vi "Measurement UI.vi"() -> ()   [LabVIEW 2021, in "Ramp-Up Time_PMIC_UI.lvlib"]
uses:
  Ramp-Up Time_PMIC_UI.lvlib
panel:
  in  "MeasGraphs":T1(tab)
  out "SourceVoltageV/STimeGraph":waveform(dbl)(graph) caption="Load Transient"
  in  "SourceOutput Voltage v/s Time":string="SOURCE VOLTAGE vs TIME"
  out "OutputVoltageV/STimeGraph":waveform(dbl)(graph) caption="Load Transient"
  in  "LoadOutput Voltage v/s Time":string="LOAD VOLTAGE vs TIME"
  out "ScopeAmplitudeV/STime":waveform(dbl)(graph) caption="Load Transient"
  in  "ScopeOutput Voltage v/s Time":string="SCOPE AMPLITUDE vs TIME"
  out "Ramp stop time":dbl
  out "Ramp start time":dbl
  out "Ramp stop voltage level":dbl
  out "Ramp start voltage level":dbl
  out "Actual ramp rate":dbl
  out "Scope amplitude dt":dbl
  out "Scope amplitudes":dbl[](array[numeric])
  out "Load voltages":dbl[](array[numeric])
  out "Load voltage dt":dbl
  out "Source voltages":dbl[](array[numeric])
  out "Source voltage dt":dbl
  in  "Load resource name":string
  in  "Scope resource name":string
  in  "Source resource name":string
  in  "Source transient response":i32(ring)=1042 items=["Slow"=1041, "Normal"=1038, "Fast"=1039, "Custom"=1042]
  out "MeasTable":string[][](table)
  in  "MeasConfigurations":T2(tab)=enum."Load Config"
  in  "Source sense":i32(ring)=1009 caption="SENSE" items=["Local"=1008, "Remote"=1009]
  in  "Source ramp stop percentage(%)":dbl=90.0 caption="STOP RAMP MEASUREMENT" format="%#_6p%"
  in  "Source ramp start percentage(%)":dbl=10.0 caption="START RAMP MEASUREMENT" format="%#_6p%"
  in  "Source voltatge V2 time":dbl=0.005 caption="TIME for V1" format="%#_6ps"
  in  "Source voltage V1 time":dbl=0.005 caption="TIME for V1" format="%#_6ps"
  in  "Source voltage ramp rate":dbl=50000.0 caption="VOLTAGE RAMP RATE LIMIT" format="%#_6pV/s"
  in  "Source maximum power":dbl=300.0 caption="MAXIMUM POWER" format="%#_6pW"
  in  "Source current limit":dbl=0.25 caption="CURRENT LIMIT" format="%#_6pA"
  in  "Source voltage set point 2(V2)":dbl=20.0 caption="VOLTAGE SET POINT 2" format="%#_6pV"
  in  "Source voltage set point 1(V1)":dbl=0.1 caption="VOLTAGE SET POINT 1" format="%#_6pV"
  in  "PPSResourceName":refnum<k15> caption="RESOURCE NAME"
  in  "Source voltage pole-zero ratio":dbl=2.0 caption="POLE-ZERO RATIO"
  in  "Source voltage gain bandwidth":dbl=2000.0 caption="GAIN BANDWIDTH" format="%#_6pHz"
  in  "Source voltage compensation frequency":dbl=3530.0 caption="COMP. FREQUENCY" format="%#_6pHz"
  in  "Source fast":bool
  in  "Source normal":bool
  in  "Source slow":bool
  in  "Source SourceAdapt":string="Voltage SourceAdapt Parameters"
  in  "Source sample rate":dbl=1800000.0 caption="SAMPLE RATE" format="%#_6pS/s"
  in  "Load current level range":dbl=4.0 caption="CURRENT LEVEL RANGE" format="%#_6pA"
  in  "Load sense":i32(ring)=1009 caption="SENSE" items=["Local"=1008, "Remote"=1009]
  in  "ELOADResourceName":refnum<k15> caption="RESOURCE NAME"
  in  "Load current level":dbl=1.0 caption="CURRENT  LEVEL" format="%#_6pA"
  in  "Load voltage limit range":dbl=6.0 caption="VOLTAGE LIMIT RANGE" format="%#_6pV"
  in  "Load enable/disable":bool caption="Load Enable/Disable"
  out "Load status":string="Load is disabled"
  in  "Load source delay":dbl=0.005 caption="SOURCE DELAY" format="%#_6ps"
  in  "Scope vertical range":dbl=10.0 caption="VERTICAL RANGE"
  out "Scope status":string="Scope is disabled"
  in  "Scope enable/disable":bool caption="Scope Enable/Disable"
  in  "SCOPEResourceName":refnum<k15> caption="RESOURCE NAME"
  in  "Scope probe attenuation":dbl=1.0 caption="PROBE ATTENUATION"
  in  "Scope sample rate":dbl=1800000.0 caption="SAMPLE RATE" format="%#_6pHz"
  in  "Scope output channel name":string="0" caption="INPUT CHANNEL NAME"
  in  "Scope vertical coupling":enum32{"AC", "DC"}(ring)=enum."DC" caption="VERTICAL COUPLING"
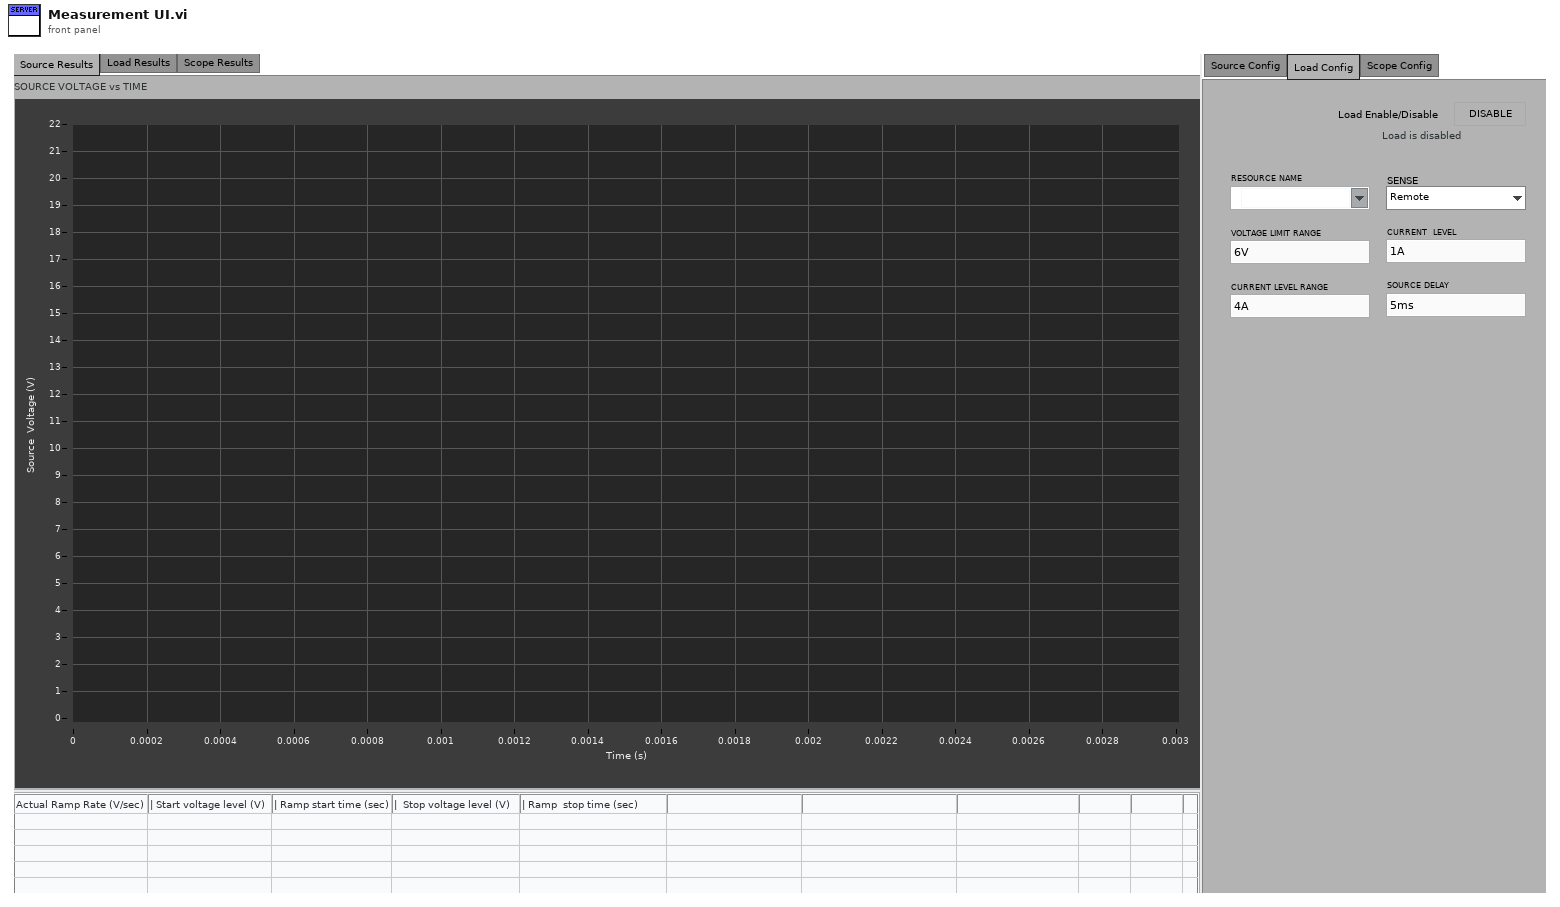
[diagram p1: front panel]
types:
  T1 = enum32{"Source Results", "Load Results", "Scope Results", "Hidden Controls"}
  T2 = enum32{"Source Config", "Load Config", "Scope Config"}
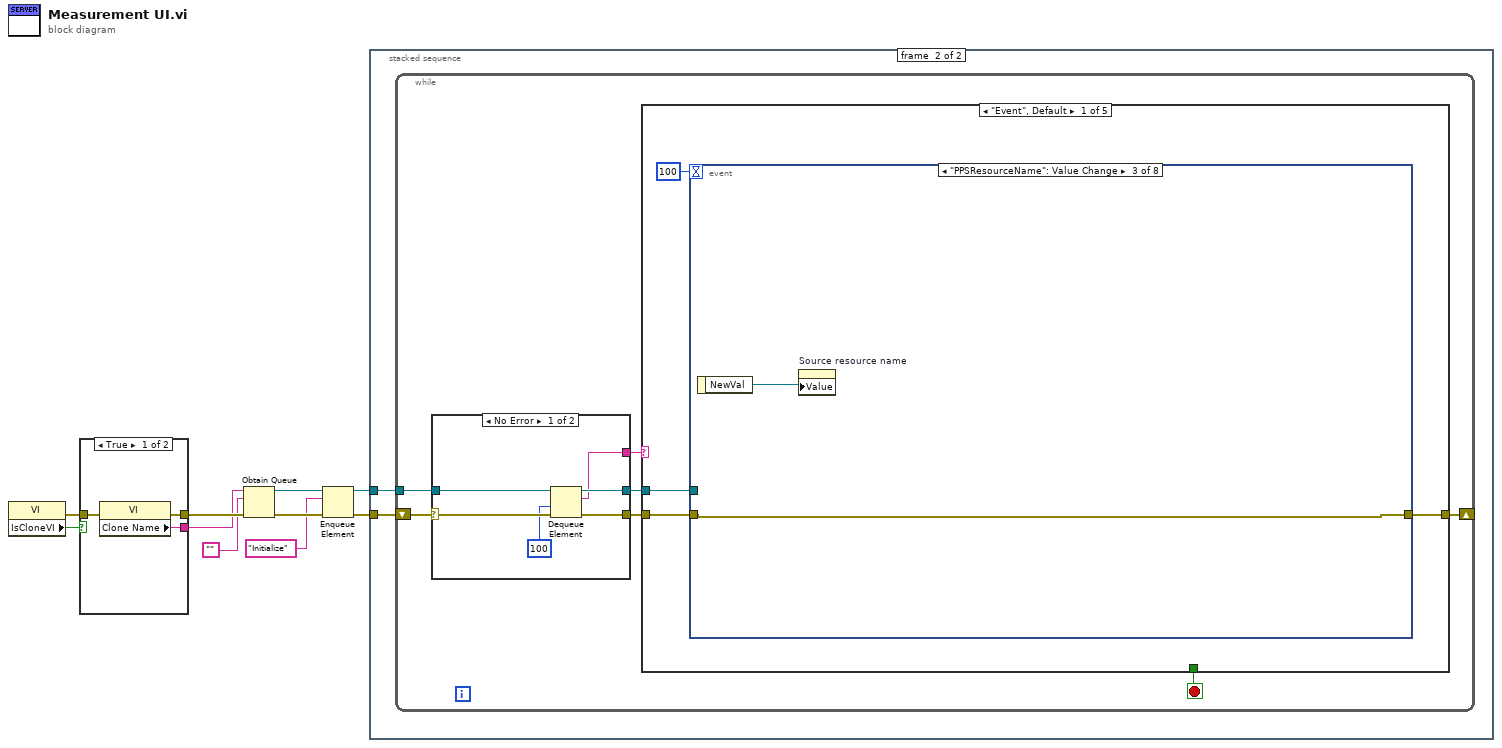
[diagram p0: block diagram]
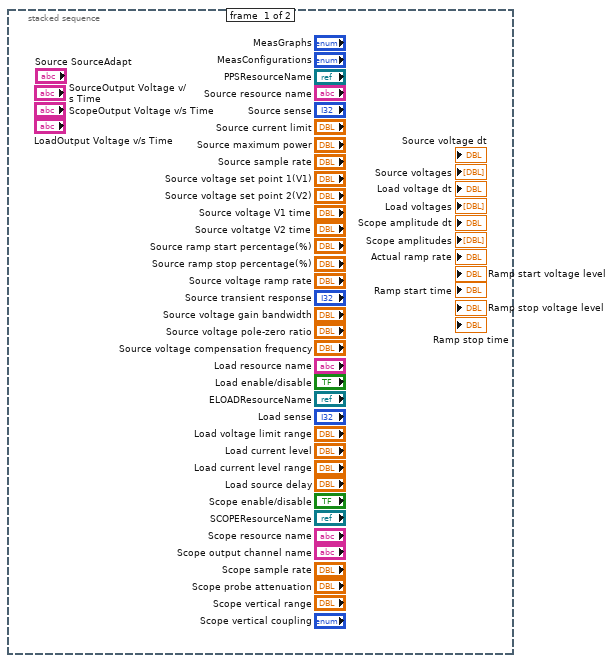
[diagram p2: hidden frame]
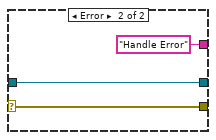
[diagram p3: hidden frame]
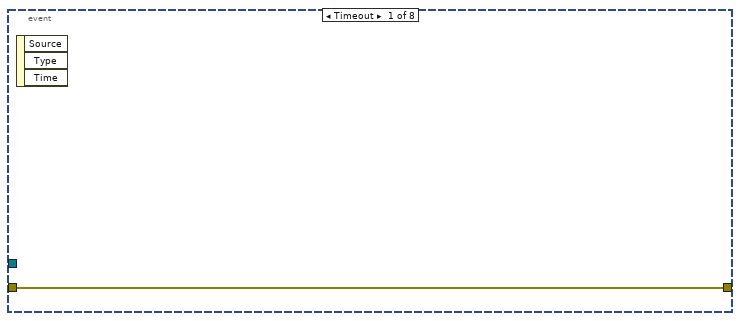
[diagram p4: hidden frame]
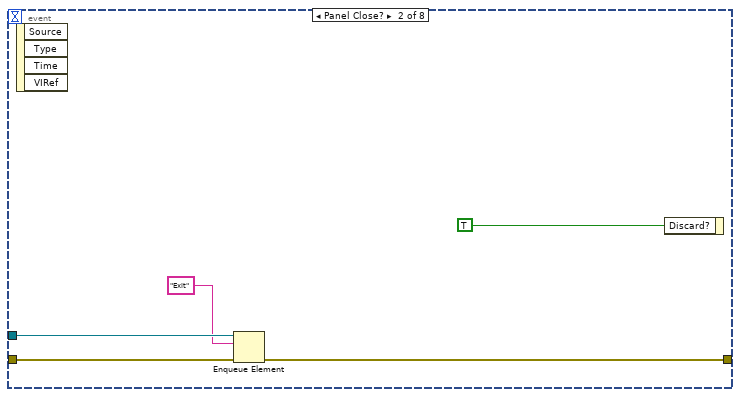
[diagram p5: hidden frame]
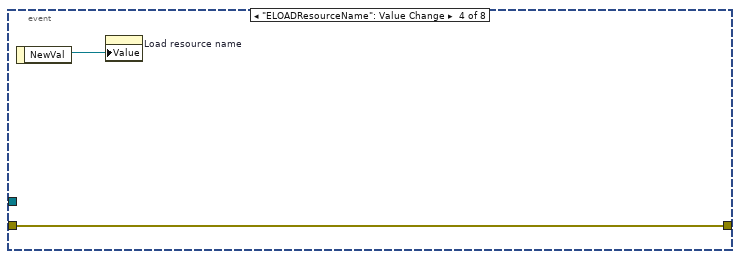
[diagram p6: hidden frame]
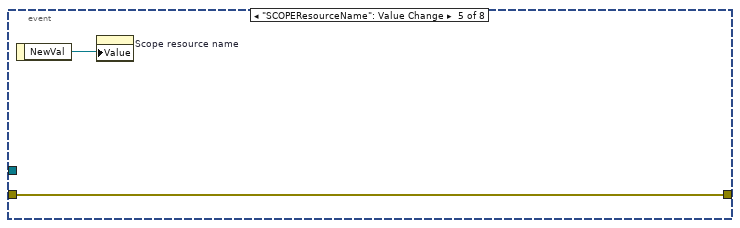
[diagram p7: hidden frame]
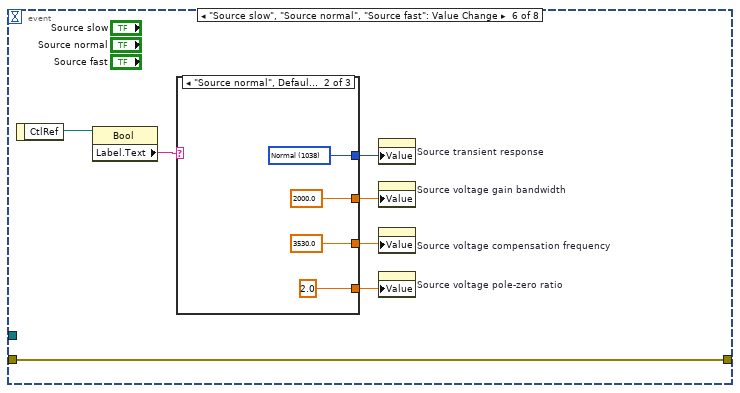
[diagram p8: hidden frame]
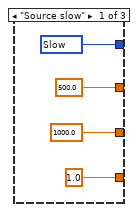
[diagram p9: hidden frame]
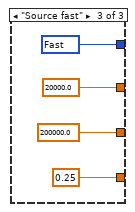
[diagram p10: hidden frame]
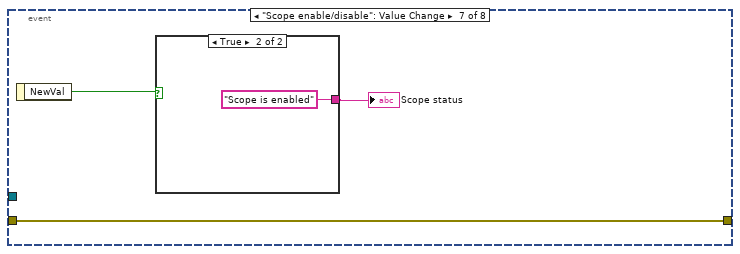
[diagram p11: hidden frame]
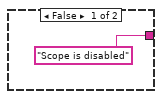
[diagram p12: hidden frame]
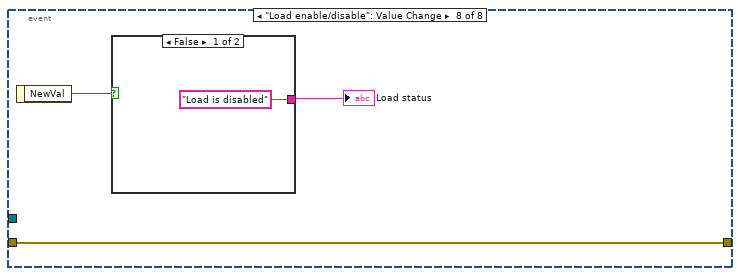
[diagram p13: hidden frame]
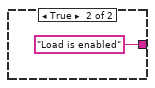
[diagram p14: hidden frame]
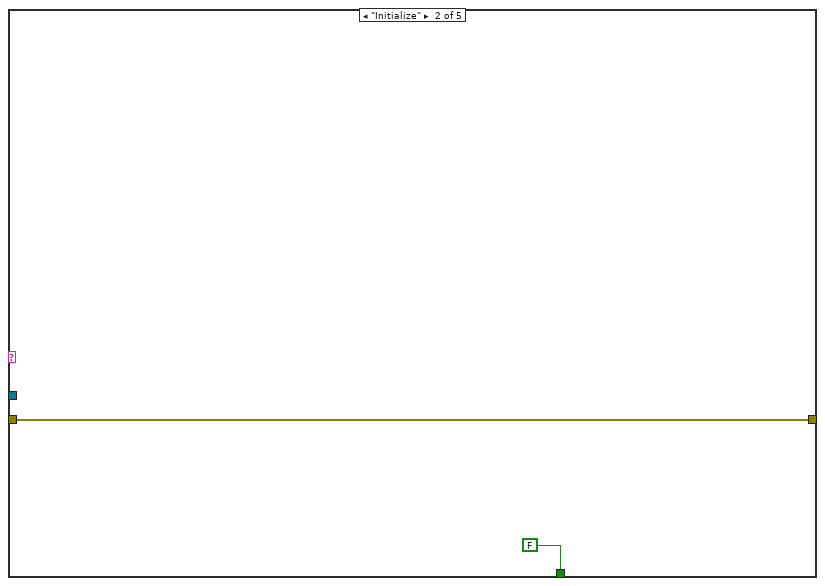
[diagram p15: hidden frame]
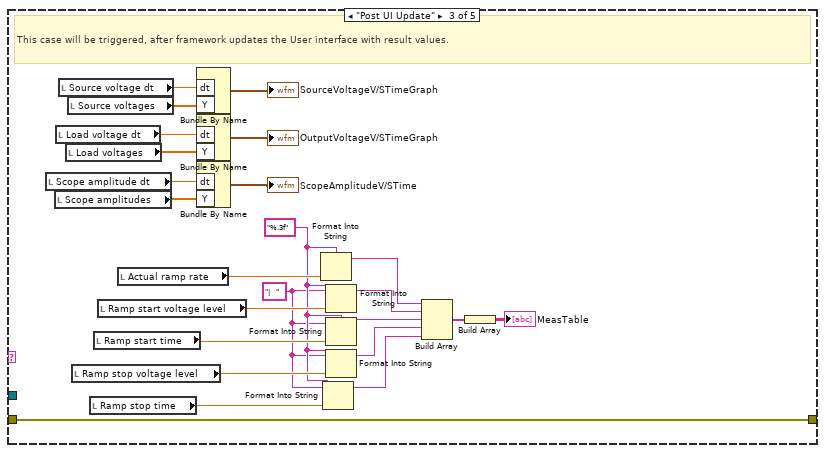
[diagram p16: hidden frame]
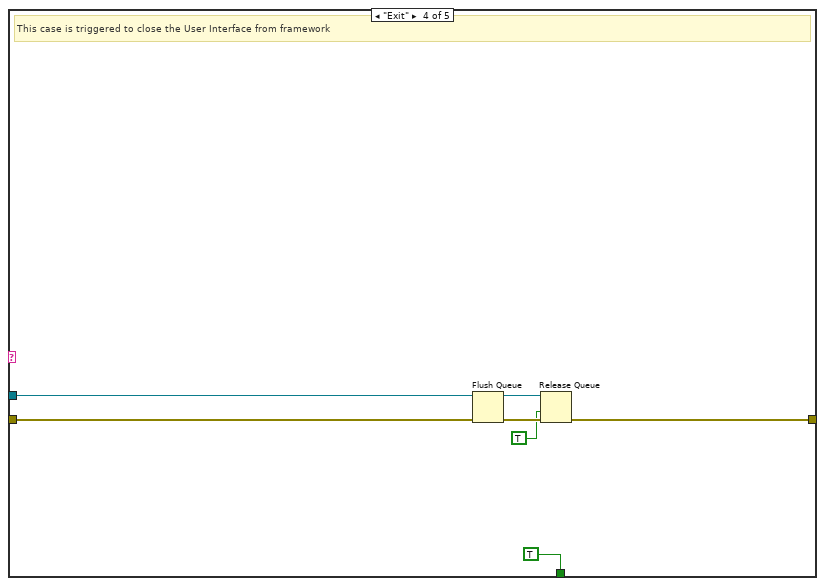
[diagram p17: hidden frame]
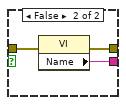
[diagram p19: hidden frame]
diagram:
  n1 = property class="VI"() -> (error out=w1:errorcluster, "IsCloneVI"=w2:bool)  [unwired: 2 in, 1 out]
  n2 = case shown="True" w2 {
    tunnel: [w13 w16] -> w10
    tunnel: [w12 w15] -> w9
    tunnel: w1 -> [w11 w14]
    frame True {
      n3 = property class="VI"(error in=w11) -> (error out=w13:errorcluster, "Clone Name"=w12:string)  [unwired: 1 in, 1 out]
    }
    frame False {
      n4 = property class="VI"(error in=w14) -> (error out=w16:errorcluster, "Name"=w15:string)  [unwired: 1 in, 1 out]
    }
  }
  n5 = Obtain Queue(name (unnamed)=w9, element data type="", error in (no error)=w10) -> (queue out=w6:refnum<queue>, error out=w8:errorcluster)  [unwired: 2 in, 1 out]
  n6 = Enqueue Element(queue=w6, element="Initialize", error in (no error)=w8) -> (queue out=w5:refnum<queue>, error out=w7:errorcluster)  [unwired: 1 in, 1 out]
  n7 = stacked-sequence {
    tunnel: w7 -> [_ w18]
    tunnel: w5 -> [_ w17]
    frame #0 {
    }
    frame #1 {
      n8 = while {
        shift-right: [w20] -> _
        shift-left: w18 -> [w25]
        tunnel: w17 -> [w23]
        stop <- w19 stop-if-true
        n9 = case shown="No Error" w25 {
          selector: w25 -> [w31 w34]
          tunnel: [w30 w34] -> w24
          tunnel: w23 -> [w29 w33]
          tunnel: [w28 w33] -> w22
          tunnel: [w27 "Handle Error"] -> w21
          frame No Error {
            n10 = Dequeue Element(queue=w29, timeout in ms (-1)=100, error in (no error)=w31) -> (queue out=w28:refnum<queue>, element=w27:string, error out=w30:errorcluster)  [unwired: 1 out]
          }
          frame Error {
          }
        }
        n11 = case shown="\"Event\", Default" w21 {
          tunnel: w24 -> [w37 w81 w105 w112 w113]
          tunnel: w22 -> [w35 _ _ w110 _]
          tunnel: [w38 w81 w105 w107 w113] -> w20
          tunnel: [_ FALSE _ TRUE _] -> w19
          frame "Event", Default {
            n12 = event shown="[2] \"PPSResourceName\": Value Change" {
              selector: _ -> [_ _ _ _ _ _ _ _]
              dyn-events: _ -> [_ _ _ _ _ _ _ _]
              timeout: 100 -> [_ _ _ _ _ _ _ _]
              tunnel: [w39 w42 w45 w47 w49 w51 w70 w75] -> w38
              tunnel: w37 -> [w39 w43 w45 w47 w49 w51 w70 w75]
              tunnel: w35 -> [_ w41 _ _ _ _ _ _]
              event Timeout {
                n13 = event-data() -> ()  [unwired: 1 in, 3 out]
              }
              event Panel Close? {
                n14 = event-data() -> ()  [unwired: 1 in, 4 out]
                n15 = Enqueue Element(queue=w41, element="Exit", error in (no error)=w43) -> (error out=w42:errorcluster)  [unwired: 1 in, 2 out]
                n16 = event-data("Discard?"=TRUE) -> ()  [unwired: 1 in, 1 out]
              }
              event "PPSResourceName": Value Change {
                n17 = event-data() -> ("NewVal"=w46:refnum<k15>)  [unwired: 1 in]
                n18 = property on="Source resource name" class="Str"("Value"=w46) -> ()  [unwired: 2 in, 2 out]
              }
              event "ELOADResourceName": Value Change {
                n19 = event-data() -> ("NewVal"=w48:refnum<k15>)  [unwired: 1 in]
                n20 = property on="Load resource name" class="Str"("Value"=w48) -> ()  [unwired: 2 in, 2 out]
              }
              event "SCOPEResourceName": Value Change {
                n21 = event-data() -> ("NewVal"=w50:refnum<k15>)  [unwired: 1 in]
                n22 = property on="Scope resource name" class="Str"("Value"=w50) -> ()  [unwired: 2 in, 2 out]
              }
              event "Source slow", "Source normal", "Source fast": Value Change {
                n23 = event-data() -> ("CtlRef"=w57:refnum<vi>)  [unwired: 1 in]
                n24 = property class="Bool"(reference=w57) -> ("Label.Text"=w56:string)  [unwired: 1 in, 2 out]
                n25 = case shown="\"Source normal\", Default" w56 {
                  tunnel: [w61 w65 w69] -> w55
                  tunnel: [500.0 ("Source voltage gain bandwidth") 2000.0 ("Source voltage gain bandwidth") 20000.0 ("Source voltage gain bandwidth")] -> w54
                  tunnel: [1000.0 ("Source voltage compensation frequency") 3530.0 ("Source voltage compensation frequency") 200000.0 ("Source voltage compensation frequency")] -> w52
                  tunnel: [1.0 ("Source voltage pole-zero ratio") 2.0 ("Source voltage pole-zero ratio") 0.25 ("Source voltage pole-zero ratio")] -> w53
                  frame "Source slow" {
                    w61 = 1041 items=["Slow"=1041, "Normal"=1038, "Fast"=1039, "Custom"=1042] ("Source transient response")
                  }
                  frame "Source normal", Default {
                    w65 = 1038 items=["Slow"=1041, "Normal"=1038, "Fast"=1039, "Custom"=1042] ("Source transient response")
                  }
                  frame "Source fast" {
                    w69 = 1039 items=["Slow"=1041, "Normal"=1038, "Fast"=1039, "Custom"=1042] ("Source transient response")
                  }
                }
                n26 = property on="Source transient response" class="Ring (strict)"("Value"=w55) -> ()  [unwired: 2 in, 2 out]
                n27 = property on="Source voltage gain bandwidth" class="DigNum (strict)"("Value"=w54) -> ()  [unwired: 2 in, 2 out]
                n28 = property on="Source voltage compensation frequency" class="DigNum (strict)"("Value"=w52) -> ()  [unwired: 2 in, 2 out]
                n29 = property on="Source voltage pole-zero ratio" class="DigNum (strict)"("Value"=w53) -> ()  [unwired: 2 in, 2 out]
              }
              event "Scope enable/disable": Value Change {
                n30 = event-data() -> ("NewVal"=w72:bool)  [unwired: 1 in]
                n31 = case shown="True" w72 {
                  tunnel: ["Scope is disabled" ("Load status") "Scope is enabled" ("Load status")] -> w71
                  frame False {
                  }
                  frame True {
                  }
                }
                "Scope status" <- w71
              }
              event "Load enable/disable": Value Change {
                n32 = event-data() -> ("NewVal"=w77:bool)  [unwired: 1 in]
                n33 = case shown="False" w77 {
                  tunnel: ["Load is disabled" ("Load status") "Load is enabled" ("Load status")] -> w76
                  frame False {
                  }
                  frame True {
                  }
                }
                "Load status" <- w76
              }
            }
          }
          frame "Initialize" {
          }
          frame "Post UI Update" {
            w83 = "%.3f" ("initial string")
            w82 = "|   " ("initial string")
            # "This case will be triggered, after framework updates the User interface with result values."
            n34 = local read "Scope amplitude dt"() -> (w102:dbl)
            n35 = local read "Scope amplitudes"() -> (w101:dbl[])
            n36 = local read "Load voltage dt"() -> (w98:dbl)
            n37 = local read "Source voltage dt"() -> (w100:dbl)
            n38 = local read "Load voltages"() -> (w97:dbl[])
            n39 = local read "Source voltages"() -> (w99:dbl[])
            n40 = local read "Ramp stop voltage level"() -> (w87:dbl)
            n41 = local read "Ramp stop time"() -> (w86:dbl)
            n42 = local read "Ramp start time"() -> (w88:dbl)
            n43 = local read "Ramp start voltage level"() -> (w89:dbl)
            n44 = local read "Actual ramp rate"() -> (w95:dbl)
            n45 = Bundle By Name("dt"=w100, "Y"=w99) -> (→"SourceVoltageV/STimeGraph":waveform(dbl))  [unwired: 1 in]
            n46 = Bundle By Name("dt"=w98, "Y"=w97) -> (→"OutputVoltageV/STimeGraph":waveform(dbl))  [unwired: 1 in]
            n47 = Bundle By Name("dt"=w102, "Y"=w101) -> (→"ScopeAmplitudeV/STime":waveform(dbl))  [unwired: 1 in]
            n48 = Format Into String(format string=w83, w95) -> (resulting string=w94:string)  [unwired: 2 in, 1 out]
            n49 = Format Into String(format string=w83, initial string=w82, w86) -> (resulting string=w85:string)  [unwired: 1 in, 1 out]
            n50 = Format Into String(format string=w83, initial string=w82, w89) -> (resulting string=w93:string)  [unwired: 1 in, 1 out]
            n51 = Format Into String(format string=w83, initial string=w82, w88) -> (resulting string=w92:string)  [unwired: 1 in, 1 out]
            n52 = Format Into String(format string=w83, initial string=w82, w87) -> (resulting string=w91:string)  [unwired: 1 in, 1 out]
            n53 = Build Array(w94, w93, w92, w91, w85) -> (w90:string[])
            n54 = Build Array(w90) -> (→"MeasTable":string[][])
          }
          frame "Exit" {
            # "This case is triggered to close the User Interface from framework"
            n55 = Flush Queue(queue=w110, error in (no error)=w112) -> (queue out=w109:refnum<queue>, error out=w108:errorcluster)  [unwired: 1 out]
            n56 = Release Queue(queue=w109, force destroy? (F)=TRUE, error in (no error)=w108) -> (error out=w107:errorcluster)  [unwired: 2 out]
          }
          frame "Handle Error" {
          }
        }
      }
    }
  }
